vi "Initialize.vi"(7 "Channel Name":string="Setpoint.ch%d.SP", 8 "error in":errorcluster, 9 "Number of Channels":u32=1, 10 "Instance Name":string="PluginName", 11 "Pressure Gradient in":refnum<class "Pressure Gradient.lvclass">) -> (0 "error out":errorcluster, 3 "Pressure Gradient out":refnum<class "Pressure Gradient.lvclass">)   [LabVIEW 2023, in "Pressure Gradient.lvclass"]
uses:
  Pressure Gradient.lvclass
  Parents/Gradient/Gradient.lvclass
  Pressure Gradient.lvclass/Pressure Gradient.ctl
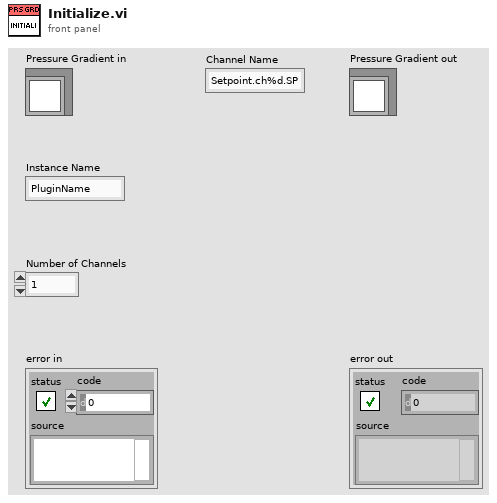
[diagram p1: front panel]
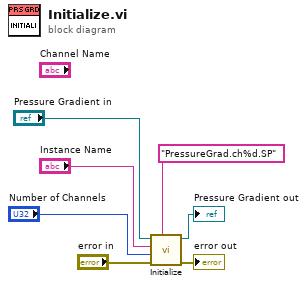
[diagram p0: block diagram]
diagram:
  n1 = call-parent "Initialize.vi"("Channel Name"="PressureGrad.ch%d.SP", "error in"="error in", "Number of Channels"="Number of Channels", "Instance Name"="Instance Name", "Gradient in"="Pressure Gradient in") -> ("error out"=→"error out":errorcluster, "Gradient out"=→"Pressure Gradient out":refnum<class "Pressure Gradient.lvclass">)  [unwired: 5 in]
